vi "LWXPS_PositionerEncoderAmplitudeValuesGet.vi"(0 "XPS Reference IN":refnum<k24>, 2 "Positioner Name":string, 5 "LabVIEW error IN":errorcluster) -> (12 "XPS Reference OUT":refnum<k24>, 13 "LabVIEW error OUT":errorcluster, 14 "Returned error code":i32, 15 "Calibration Sinus Amplitude":dbl, 16 "Current Sinus Amplitude":dbl, 17 "Calibration Cosinus Amplitude":dbl, 18 "Current Cosinus Amplitude":dbl, 19 "XPS Error String":string)   [LabVIEW 2014]
uses:
  D:/XPSQ8_LabView_Library/Development/Source/Dll/Newport.XPS.CommandInterface.dll
  Dll/Newport.XPS.CommandInterface.dll
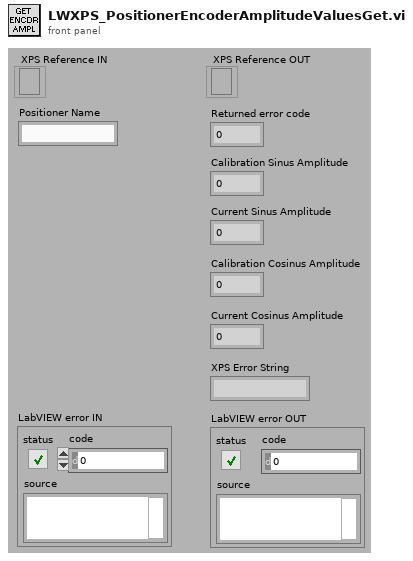
[diagram p1: front panel]
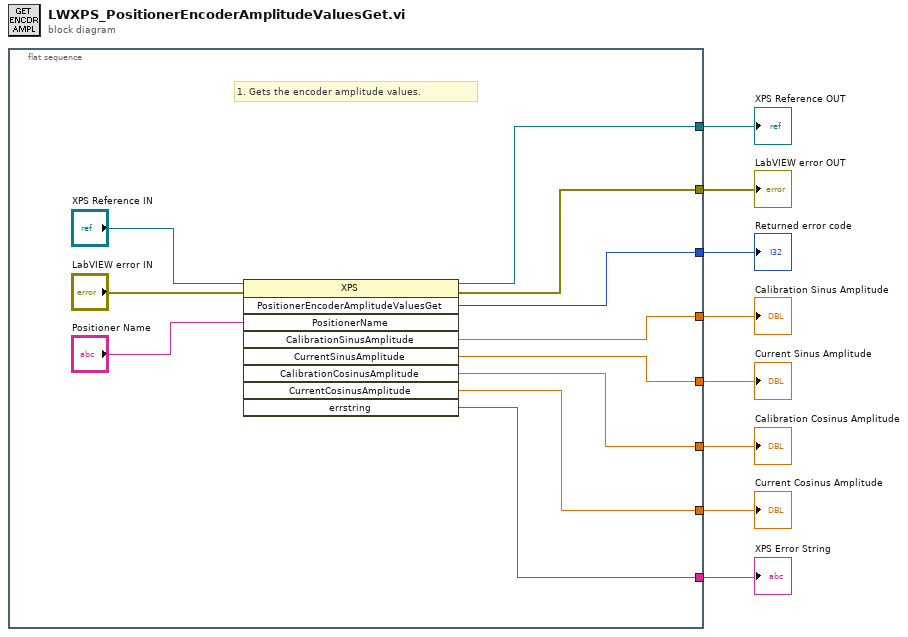
[diagram p0: block diagram]
diagram:
  n1 = flat-sequence {
    tunnel: [w17] -> w8
    tunnel: [w14] -> w7
    tunnel: [w18] -> w6
    tunnel: [w9] -> w1
    tunnel: [w13] -> w5
    tunnel: [w12] -> w4
    tunnel: [w11] -> w2
    tunnel: [w10] -> w3
    frame #0 {
      # "1. Gets the encoder amplitude values."
      n2 = invoke class="XPS" method="PositionerEncoderAmplitudeValuesGet"(reference="XPS Reference IN", error in="LabVIEW error IN", "PositionerName"="Positioner Name") -> (reference out=w17:refnum<k24>, error out=w14:errorcluster, "PositionerEncoderAmplitudeValuesGet"=w18:i32, "CalibrationSinusAmplitude"=w9:dbl, "CurrentSinusAmplitude"=w13:dbl, "CalibrationCosinusAmplitude"=w12:dbl, "CurrentCosinusAmplitude"=w11:dbl, "errstring"=w10:string)  [unwired: 6 in, 1 out]
    }
  }
  "XPS Error String" <- w3
  "XPS Reference OUT" <- w8
  "LabVIEW error OUT" <- w7
  "Returned error code" <- w6
  "Current Sinus Amplitude" <- w5
  "Calibration Cosinus Amplitude" <- w4
  "Current Cosinus Amplitude" <- w2
  "Calibration Sinus Amplitude" <- w1
